vi "population_container.vi"(0 "Thermally Connect Zero Ensemble":bool, 1 "Microwave on":bool, 2 "Zero Level on":bool, 3 "Zero Ensemble Area":dbl, 4 "RF Indicator":bool, 5 "Normed Array 2":dbl[](array[numeric]), 6 "Zero Ensemble Power":dbl, 8 "Drive Zero Level Down":bool, 9 "Normed Array 3":dbl[](array[numeric]), 10 "RF Power":dbl, 11 "Relaxation Rate":dbl, 12 "AFP Efficiency":dbl, 13 "Microwave Power":dbl, 14 "Numeric 2":i32, 15 "Array":dbl[](array[numeric]), 16 "Numeric":i32, 17 "Array 2":dbl[](array[numeric]), 18 "RF Proportional to Intensity":bool, 19 "Array 4":dbl[](array[numeric]), 25 "Normed Array":dbl[](array[numeric]), 26 "Array 3":dbl[](array[numeric]), 27 "Saturation Polarization":dbl) -> (20 "Zero ensemble out":dbl[](array[numeric]), 21 "rho- out":dbl[](array[numeric]), 22 "rho+ out":dbl[](array[numeric]), 23 "rho0 out":dbl[](array[numeric]))   [LabVIEW 2018]
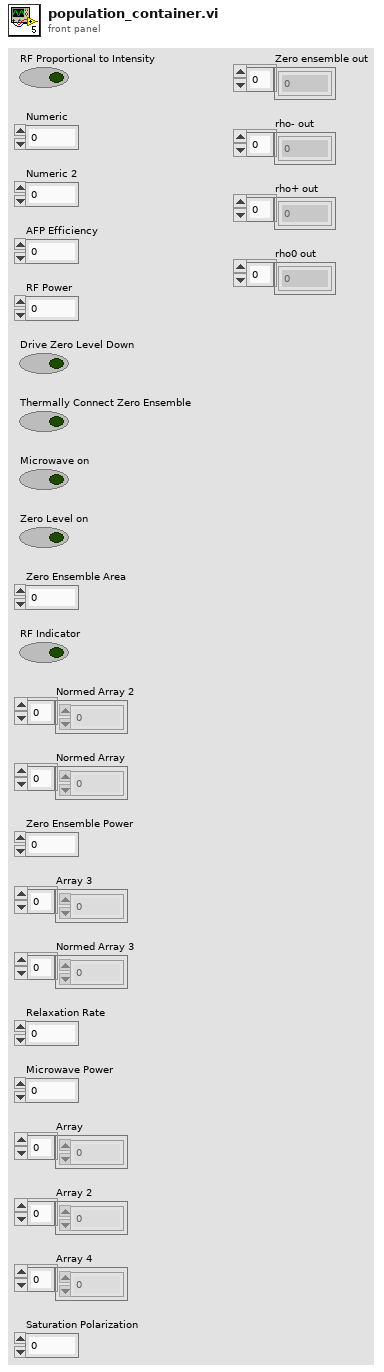
[diagram p1: front panel]
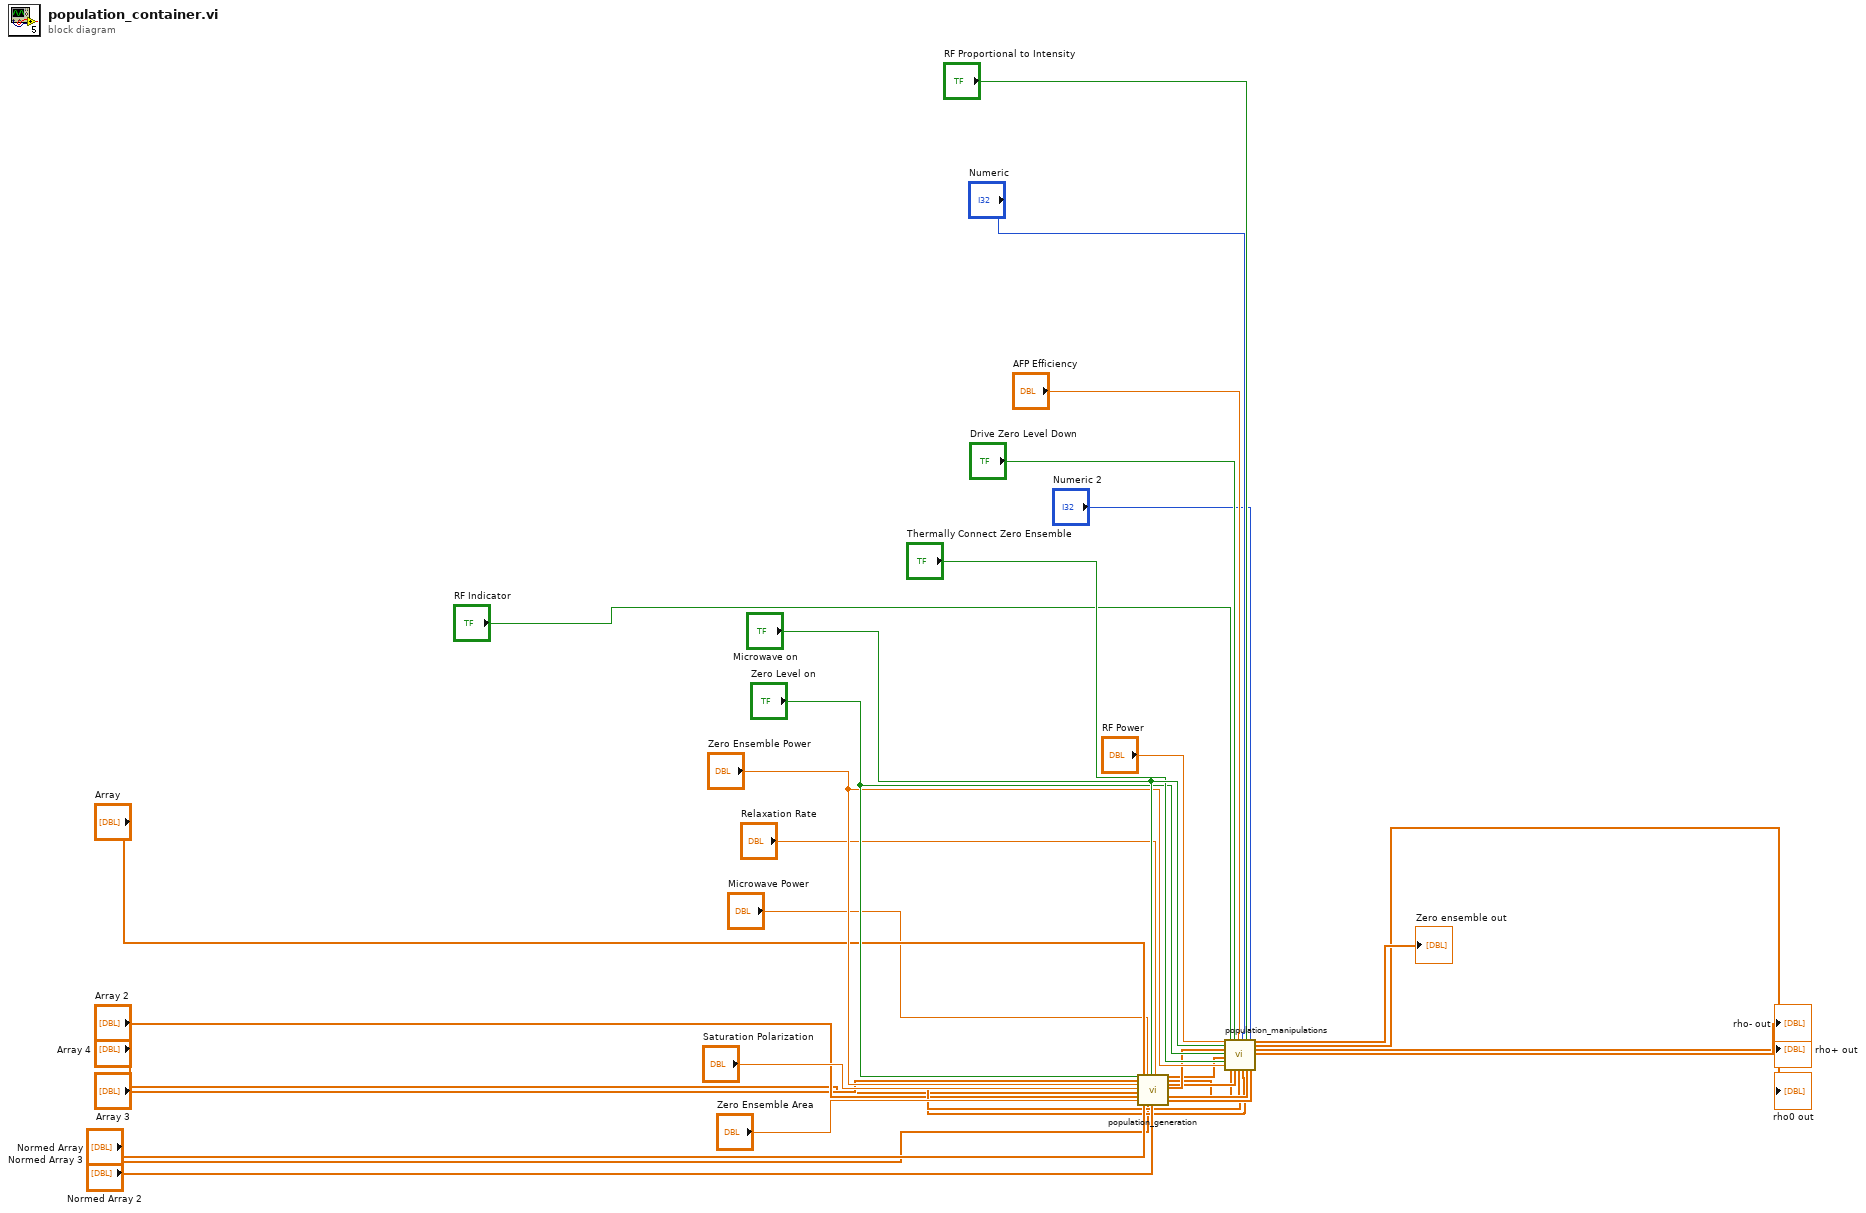
[diagram p0: block diagram]
diagram:
  n1 = call "population_generation.vi"("Zero Level on"="Zero Level on", "Array 3"="Array 3", "Zero Ensemble Power"="Zero Ensemble Power", "Saturation Polarization"="Saturation Polarization", "Array 4"="Array 4", "Array 2"="Array 2", "Zero Ensemble Area"="Zero Ensemble Area", "Array"="Array", "Normed Array"="Normed Array", "Microwave Power"="Microwave Power", "Normed Array 3"="Normed Array 3", "Microwave on"="Microwave on", "Normed Array 2"="Normed Array 2", "Relaxation Rate"="Relaxation Rate") -> ("Zero Ensemble Out"=w26:dbl[], "rho- array out 2"=w10:dbl[], "rho+ array out"=w13:dbl[], "rho0 array out 2"=w14:dbl[], "rho- array out"=w15:dbl[], "rho+ array out 2"=w11:dbl[], "rho0 array out"=w24:dbl[], "rho0 decay out"=w25:dbl[])  [unwired: 6 in]
  n2 = call "population_manipulations.vi"("RF Power"="RF Power", "Microwave on"="Microwave on", "Zero Ensemble Out"=w26, "Zero Level on"="Zero Level on", 4:"rho- array in"=w10, "Thermally Connect Zero Ensemble"="Thermally Connect Zero Ensemble", "Zero Ensemble Power"="Zero Ensemble Power", "RF Indicator"="RF Indicator", 9:"rho+ array in"=w13, "Drive Zero Level Down"="Drive Zero Level Down", 11:"rho0 array in"=w14, "AFP Efficiency"="AFP Efficiency", 13:"rho- array in"=w15, "Numeric"="Numeric", 15:"rho+ array in"=w11, "RF Proportional to Intensity"="RF Proportional to Intensity", 17:"rho0 array in"=w24, "Numeric 2"="Numeric 2", "rho0 decay in"=w25) -> ("Zero ensemble out"=→"Zero ensemble out":dbl[], "rho0 out"=→"rho0 out":dbl[], "rho+ out"=→"rho+ out":dbl[], "rho- out"=→"rho- out":dbl[])  [unwired: 5 in]
